vi "Periodic Tasks.vi"(8 "error in":errorcluster) -> ()   [LabVIEW 2016]
doc: "This VI runs in parallel to other tasks. It can contain as many user-defined periodic loops as you need. These can carry out PID or other sorts of timed response."
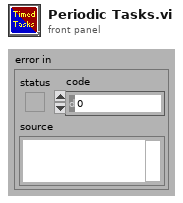
[diagram p1: front panel]
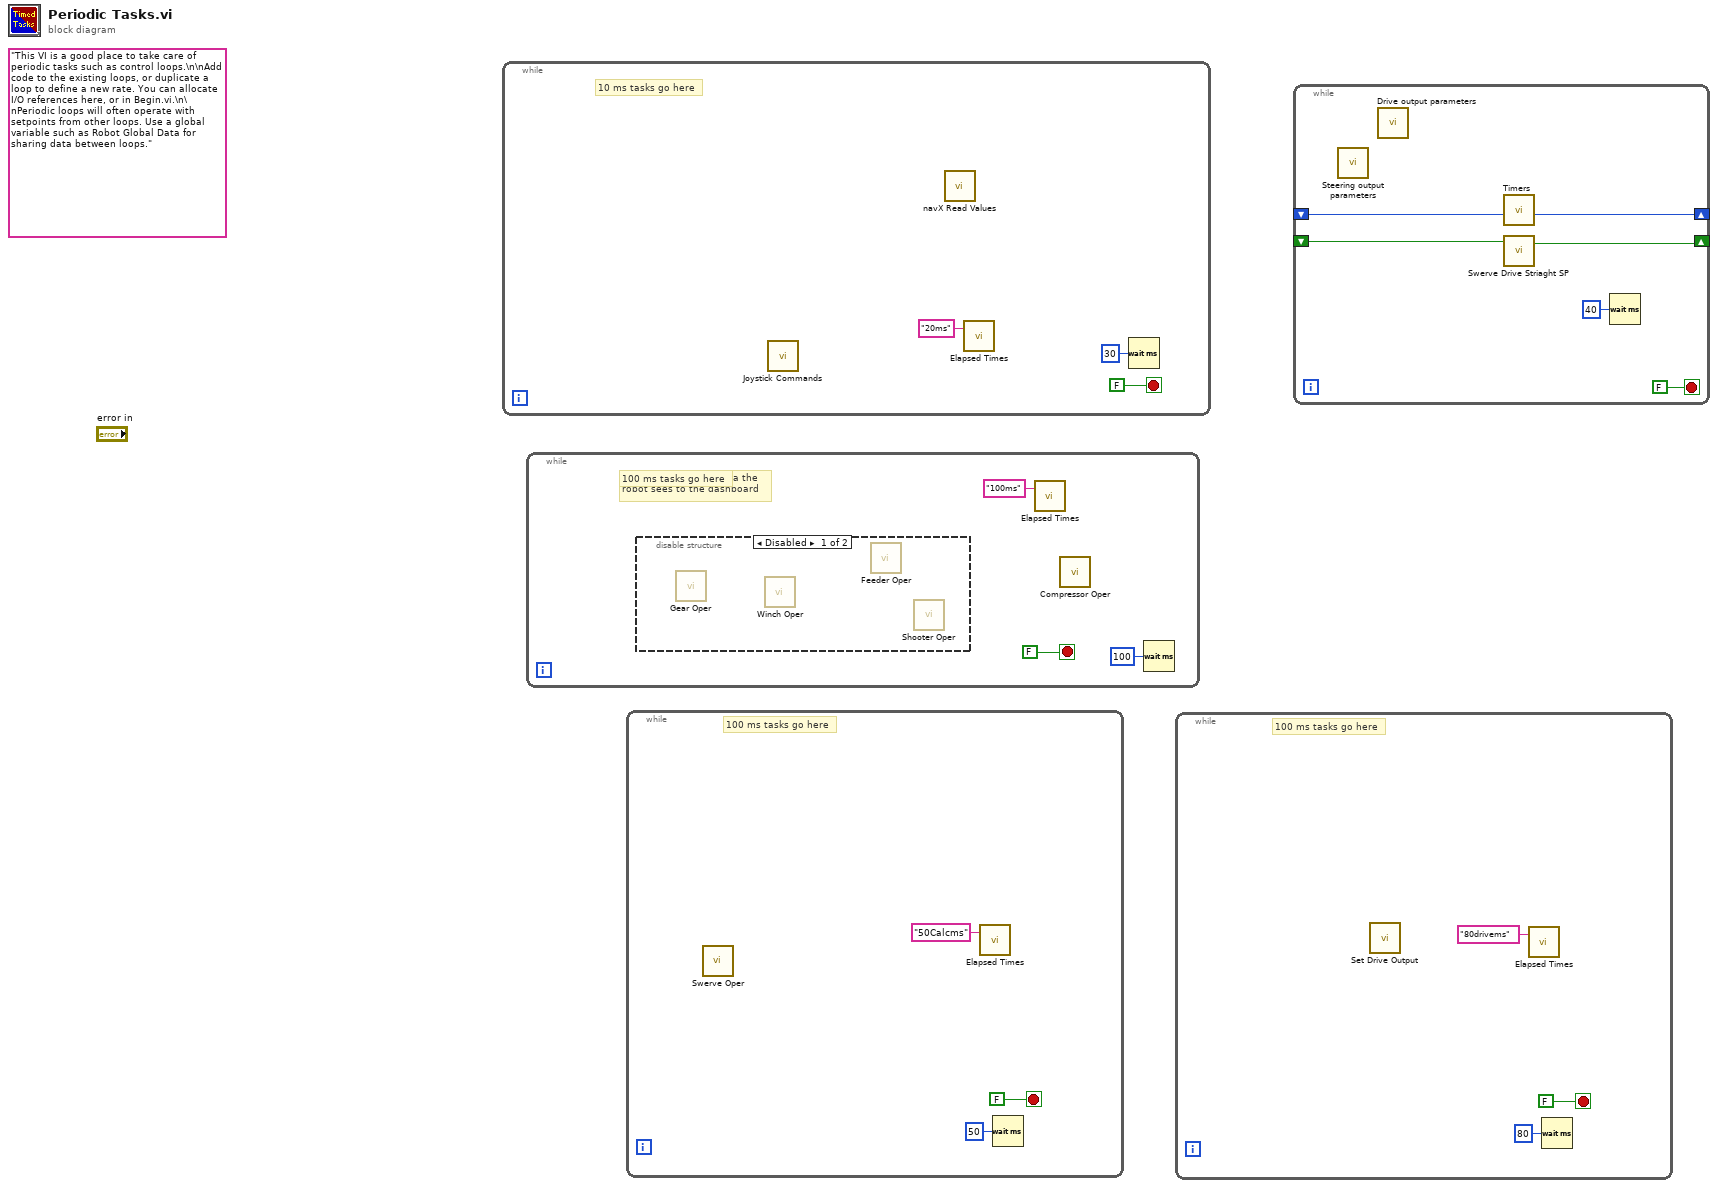
[diagram p0: block diagram]
diagram:
  (unwired) "This VI is a good place to take care of periodic tasks such as control loops.\n\nAdd code to the existing loops, or duplicate a loop to define a new rate. You can allocate I/O references here, or in Begin.vi.\n\nPeriodic loops will often operate with setpoints from other loops. Use a global variable such as Robot Global Data for sharing data between loops."
  n1 = while {
    stop <- FALSE stop-if-true
    # "10 ms tasks go here"
    n2 = call "Joystick Commands.vi"() -> ()  [unwired: 12 in]
    n3 = call "navX Read Values.vi"() -> ()  [unwired: 2 in, 1 out]
    n4 = call "Elapsed Times.vi"("Call Name"="20ms") -> ()  [unwired: 2 in, 1 out]
    n5 = Wait (ms)(milliseconds to wait=u32 30) -> ()  [unwired: 1 out]
  }
  n6 = while {
    stop <- FALSE stop-if-true
    # "Publish the joystick data the\nrobot sees to the dashboard"
    # "100 ms tasks go here"
    n7 = disable-structure shown="Disabled" {
      frame Disabled {
        n8 = call "Gear Oper.vi"() -> ()  [unwired: 12 in]
        n9 = call "Winch Oper.vi"() -> ()  [unwired: 12 in]
        n10 = call "Feeder Oper.vi"() -> ()  [unwired: 12 in]
        n11 = call "Shooter Oper.vi"() -> ()  [unwired: 12 in]
      }
      frame Enabled {
      }
    }
    n12 = call "Elapsed Times.vi"("Call Name"="100ms") -> ()  [unwired: 2 in, 1 out]
    n13 = call "Compressor Oper.vi"() -> ()  [unwired: 12 in]
    n14 = Wait (ms)(milliseconds to wait=u32 100) -> ()  [unwired: 1 out]
  }
  n15 = while {
    stop <- FALSE stop-if-true
    # "100 ms tasks go here"
    n16 = call "Swerve Oper.vi"() -> ()  [unwired: 12 in]
    n17 = call "Elapsed Times.vi"("Call Name"="50Calcms") -> ()  [unwired: 2 in, 1 out]
    n18 = Wait (ms)(milliseconds to wait=u32 50) -> ()  [unwired: 1 out]
  }
  n19 = while {
    stop <- FALSE stop-if-true
    # "100 ms tasks go here"
    n20 = call "Set Drive Output.vi"() -> ()  [unwired: 12 in]
    n21 = call "Elapsed Times.vi"("Call Name"="80drivems") -> ()  [unwired: 2 in, 1 out]
    n22 = Wait (ms)(milliseconds to wait=u32 80) -> ()  [unwired: 1 out]
  }
  n23 = while {
    shift-right: [w16] -> _
    shift-left: _ -> [w14]
    shift-right: [w15] -> _
    shift-left: _ -> [w13]
    stop <- FALSE stop-if-true
    n24 = call "Steering output parameters.vi"() -> ()  [unwired: 12 in]
    n25 = call "Drive output parameters.vi"() -> ()  [unwired: 12 in]
    n26 = call "Timers.vi"("Timer in"=w14) -> ("Timer out"=w16:u32)  [unwired: 10 in]
    n27 = call "Swerve Drive Striaght SP.vi"("Carry In"=w13) -> ("Carry out"=w15:bool)  [unwired: 2 in]
    n28 = Wait (ms)(milliseconds to wait=u32 40) -> ()  [unwired: 1 out]
  }
